vi "通信解析数据.vi"(8 "error in (no error)":errorcluster, 10 "Buffer('')":string, 11 "串口通信类 in":refnum<class "串口通信类.lvclass">) -> (0 "error out":errorcluster, 2 "本次解析有效？":bool, 3 "串口通信类 out":refnum<class "串口通信类.lvclass">)   [LabVIEW 2015, in "串口通信类.lvclass"]
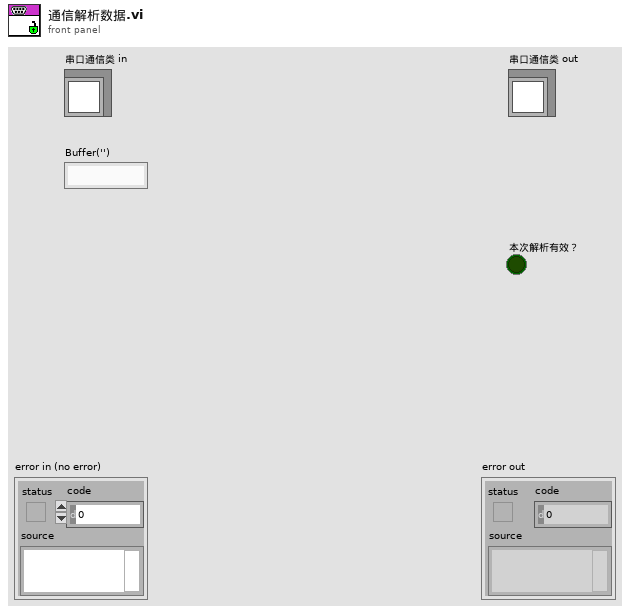
[diagram p1: front panel]
types:
  T1 = cluster{"State":string, "Data":u8[], "ID":u8, "Data Length":i32}
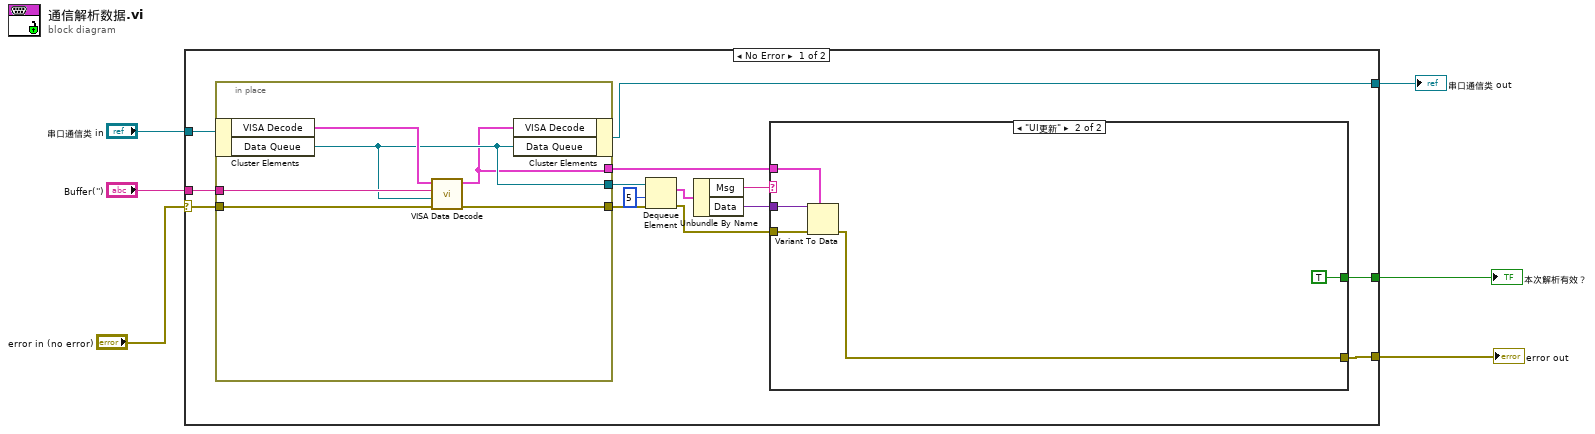
[diagram p0: block diagram]
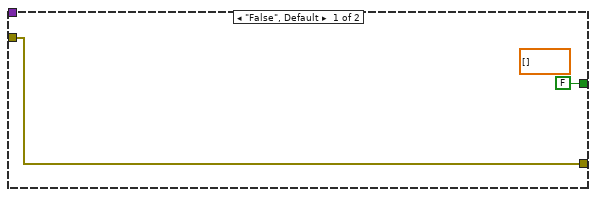
[diagram p2: hidden frame]
diagram:
  n1 = case shown="No Error" "error in (no error)" {
    selector: "error in (no error)" -> [w19 w35]
    tunnel: "串口通信类 in" -> [w20 w34]
    tunnel: "Buffer('')" -> [w18 _]
    tunnel: [w9 _] -> w3
    tunnel: [w8 w35] -> w2
    tunnel: [w7 w34] -> w1
    frame No Error {
      n2 = in-place {
        in-place-border: w19 -> [w32]
        in-place-border: w18 -> [w31]
        in-place-border: [w30] -> w16
        in-place-border: [w29] -> w17
        in-place-border: [w28] -> w11
        n3 = in-place-cluster #1(w20) -> ("VISA Decode"=w33:T1, "Data Queue"=w29:refnum<queue>)
        n4 = call "VISA Data Decode.vi"("error in (no error)"=w32, "UI Q"=w29, "Msg"=w31, "VISA Decode"=w33) -> ("error out"=w30:errorcluster, "VISA Decode out"=w28:T1)  [unwired: 6 in]
        n5 = in-place-cluster #1("VISA Decode"=w28, "Data Queue"=w29) -> (w7:refnum<class "串口通信类.lvclass">)
      }
      n6 = Dequeue Element(queue=w17, timeout in ms (-1)=5, error in (no error)=w16) -> (element=w14:cluster{"Msg":string, "Data":variant}, error out=w10:errorcluster)  [unwired: 2 out]
      n7 = Unbundle By Name(w14) -> ("Msg"=w13:string, "Data"=w12:variant)
      n8 = case shown="\"UI更新\"" w13 {
        tunnel: w12 -> [_ w27]
        tunnel: w11 -> [_ w26]
        tunnel: w10 -> [w21 w25]
        tunnel: [FALSE TRUE] -> w9
        tunnel: [w21 w23] -> w8
        frame "False", Default {
          (unwired) dbl[] []
        }
        frame "UI更新" {
          n9 = Variant To Data(error in=w25, type=w26, Variant=w27) -> (error out=w23:errorcluster)  [unwired: 1 out]
        }
      }
    }
    frame Error {
    }
  }
  "本次解析有效？" <- w3
  "error out" <- w2
  "串口通信类 out" <- w1
